vi "Toque na bola.vi"(10 "IA State":T1) -> (2 "Toque na bola ?":bool)   [LabVIEW 2016]
uses:
  Core/AI Input.ctl
  Core/AI Robot.ctl
  Intel/Functions Enum.ctl
  Core/AI Ball.ctl
  Core/Field Size.ctl
  Core/AI Judge.ctl
  Intel/Command Enum.ctl
panel:
  out "Modulo":dbl
  in  "dist para toque":dbl=130.0 format="%#_13g"
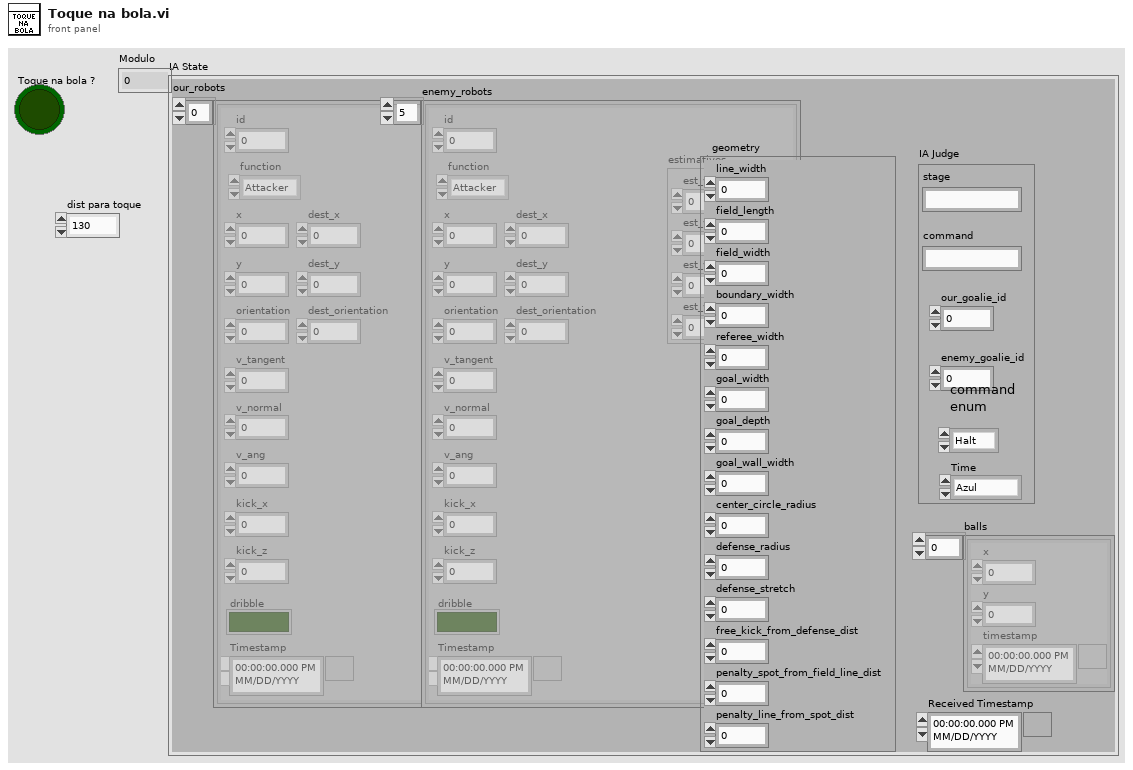
[diagram p1: front panel]
types:
  T1 = typedef "AI Input.ctl" = cluster{"our_robots":T2[], "enemy_robots":T2[], "balls":T4[], "geometry":T5, "IA Judge":T6, "Received Timestamp":timestamp}
  T2 = typedef "AI Robot.ctl" = cluster{"id":u32, "function":T3, "x":dbl, "y":dbl, "orientation":dbl, "v_tangent":dbl, "v_normal":dbl, "v_ang":dbl, "kick_x":dbl, "kick_z":dbl, "dribble":bool, "Timestamp":timestamp, "dest_x":dbl, "dest_y":dbl, "dest_orientation":dbl, "estimatives":cluster{"est_v_tangent":dbl, "est_v_normal":dbl, "est_vx":dbl, "est_vy":dbl}}
  T3 = typedef "Functions Enum.ctl" = enum16{"Attacker", "Goalie", "Defender", "Striker", "Goto 0", "Dummy", "ZigZag"}
  T4 = typedef "AI Ball.ctl" = cluster{"x":dbl, "y":dbl, "timestamp":timestamp}
  T5 = typedef "Field Size.ctl" = cluster{"line_width":u32, "field_length":u32, "field_width":u32, "boundary_width":u32, "referee_width":u32, "goal_width":u32, "goal_depth":u32, "goal_wall_width":u32, "center_circle_radius":u32, "defense_radius":u32, "defense_stretch":u32, "free_kick_from_defense_dist":u32, "penalty_spot_from_field_line_dist":u32, "penalty_line_from_spot_dist":u32}
  T6 = typedef "AI Judge.ctl" = cluster{"stage":string, "command":string, "our_goalie_id":dbl, "enemy_goalie_id":dbl, "command\nenum":T7, "Time":enum16{"Azul", "Amarelo"}}
  T7 = typedef "Command Enum.ctl" = enum16{"Halt", "Stop", "Force Start", "PKA Normal Start", "Prepare Kickoff Ally", "PKE Normal Start", "Prepare Kickoff Enemy", "Prepare Penalty Ally", "PPA Normal Start", "Prepare Penalty Enemy", "PPE Normal Start", "Direct Free Enemy", "Direct Free Ally", "Indirect Free Enemy", "Indirect Free Ally", "Timeout Enemy", "Timeout Ally", "Goal Enemy", "Goal Ally", "Ball Placement Enemy", "Ball Placement Ally", "None"}
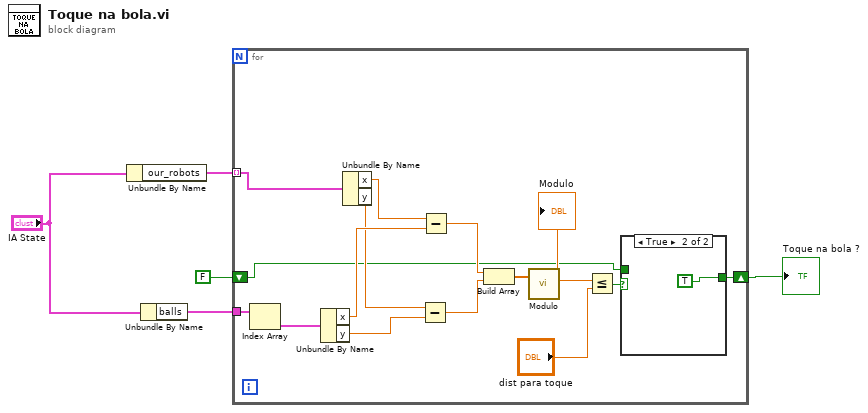
[diagram p0: block diagram]
diagram:
  n1 = Unbundle By Name("IA State") -> ("our_robots"=w5:T2[])
  n2 = Unbundle By Name("IA State") -> ("balls"=w3:T4[])
  n3 = for {
    tunnel: w5 -> [w19] mode=indexing
    tunnel: w3 -> [w20]
    shift-right: [w6] -> w2
    shift-left: FALSE -> [w7]
    n4 = Index Array(array=w20) -> (element=w18:T4)  [unwired: 1 in]
    n5 = Unbundle By Name(w18) -> ("x"=w16:dbl, "y"=w14:dbl)
    n6 = Unbundle By Name(w19) -> ("x"=w17:dbl, "y"=w11:dbl)
    n7 = Subtract(x=w11, y=w14) -> (x-y=w13:dbl)
    n8 = Subtract(x=w17, y=w16) -> (x-y=w15:dbl)
    n9 = Build Array(w15, w13) -> (w12:dbl[])
    n10 = call "Modulo.vi"("2D vector"=w12) -> ("Modulo"=w10:dbl)  [unwired: 10 in]
    "Modulo" <- w10
    n11 = Less Or Equal?(x=w10, y="dist para toque") -> (x <= y?=w8:bool)
    n12 = case shown="True" w8 {
      tunnel: w7 -> [w21 _]
      tunnel: [w21 TRUE] -> w6
      frame False {
      }
      frame True {
      }
    }
  }
  "Toque na bola ?" <- w2
